vi "fxpProperty_RoundingMode_Read.vi"(4 "error in (no error)":errorcluster, 6 "Container State":T7, 7 "Display State In":T2) -> (0 "error out":errorcluster, 2 "Value":T1, 3 "Display State Out":T2)   [LabVIEW 2020, in "FXP.xctl"]
uses:
  <vilib>/fxp/FXPxcontrol/FXP.xctl
  <vilib>/_xctls/Container State.ctl
  <vilib>/fxp/FXPxcontrol/fxpState.ctl
  <vilib>/fxp/LVFixedPointQuantizationPolicyTypeDef.ctl
  <vilib>/fxp/LVFixedPointOverflowPolicyTypeDef.ctl
  <vilib>/fxp/FXPxcontrol/fxpChangeEvent.ctl
  <vilib>/fxp/FXPxcontrol/fxpValueChangeControl.ctl
  <vilib>/fxp/FXPxcontrol/fxpMixedStateStatus.ctl
  <vilib>/_xctls/XControlSupport.lvlib
panel:
  # "Replace the Value Indicator below with an Indicator of desired type.\nDo not remove this Indicator or the others from the connector pane. \nDo not change the connector pane pattern.\nThe Value Indicator should always be the second terminal from top on the output side in the connector pane."
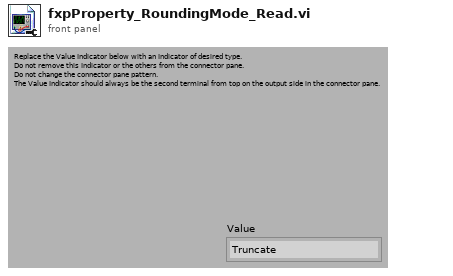
[diagram p1: front panel]
types:
  T1 = typedef "LVFixedPointQuantizationPolicyTypeDef.ctl" = enum32{"Truncate", "Round-Half-Up (Asymmetric)", "Round-Half-Even"}
  T2 = typedef "FXP.xctl/fxpState.ctl" = cluster{"disableAllConfig":bool, "disableEncodingConfig":bool, "disableRangeConfig":bool, "disableOverflowStatus":bool, "disableOverflowMode":bool, "visibleModes":bool, "visibleOverflowStatus":bool, "quantizationPolicy":T1, "overflowPolicy":T3, "includeOverflowStatus":bool, "changeEvent":T4, "valueChanged":T5, "mixed state":T6, "disableRoundingMode":bool}
  T3 = typedef "LVFixedPointOverflowPolicyTypeDef.ctl" = enum32{"Wrap", "Saturate"}
  T4 = typedef "FXP.xctl/fxpChangeEvent.ctl" = enum16{"<none>", "initialize", "modesVisible", "overflowModeEnabled", "overflowStatusVisible", "configEnabled", "modeRounding", "modeOverflow", "statusOverflow", "mixedState", "roundingModeEnabled"}
  T5 = typedef "FXP.xctl/fxpValueChangeControl.ctl" = enum16{"<none>", "sign", "word length", "integer word length", "minimum", "maximum", "delta", "rounding mode", "overflow mode", "overflow status"}
  T6 = typedef "FXP.xctl/fxpMixedStateStatus.ctl" = cluster{"sign":bool, "word length":bool, "integer word length":bool, "minimum":bool, "maximum":bool, "delta":bool, "rounding mode":bool, "overflow mode":bool, "overflow status":bool}
  T7 = typedef "XControlSupport.lvlib/Container State.ctl" = cluster{"Indicator?":bool, "Run Mode?":bool, " Refnum":refnum<vi>}
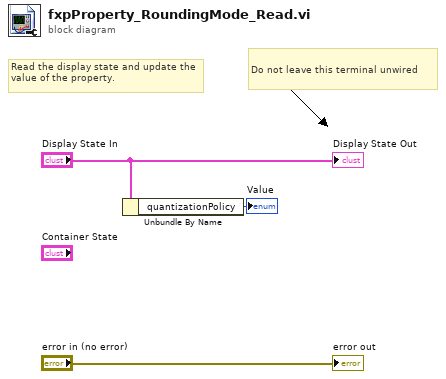
[diagram p0: block diagram]
diagram:
  # "Do not leave this terminal unwired"
  # "Read the display state and update the value of the property."
  n1 = Unbundle By Name("Display State In") -> ("quantizationPolicy"=→"Value":T1)
  "error out" <- "error in (no error)"
  "Display State Out" <- "Display State In"
